vi "Update State String.vi"(8 "error in (no error)":errorcluster, 10 "State":string, 11 "Root Actor Logic in":refnum<class "Root Actor Logic.lvclass">) -> (0 "error out":errorcluster, 3 "Root Actor Logic out":refnum<class "Root Actor Logic.lvclass">)   [LabVIEW 2021, in "Root Actor Logic.lvlib" / "Root Actor Logic.lvclass"]
uses:
  Root Actor Logic.lvclass
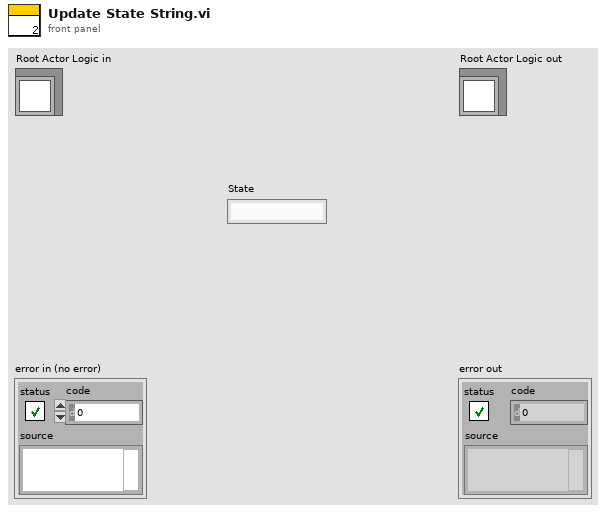
[diagram p1: front panel]
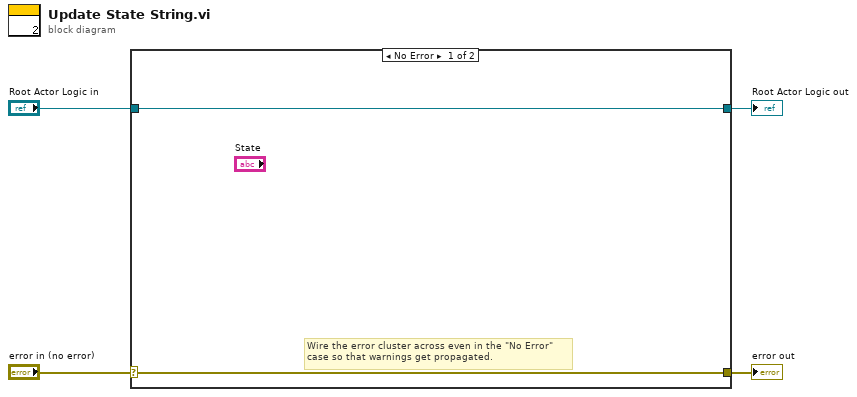
[diagram p0: block diagram]
diagram:
  n1 = case shown="No Error" "error in (no error)" {
    selector: "error in (no error)" -> [w5 w8]
    tunnel: [w5 w8] -> w3
    tunnel: [w6 w7] -> w1
    tunnel: "Root Actor Logic in" -> [w6 w7]
    frame No Error {
      # "Wire the error cluster across even in the \"No Error\"\ncase so that warnings get propagated."
    }
    frame Error {
    }
  }
  "error out" <- w3
  "Root Actor Logic out" <- w1
